vi "Format.vi"(6 "Statement":T1={"timestamp"=timestamp(0 s since 1904-01-01), "level"=enum."INFO", "sourceTag"="", "originVI"="", "message"=""}, 8 "error in (no error)":errorcluster, 11 "CSVLayout in":refnum<class "CSVLayout.lvclass">) -> (0 "error out":errorcluster, 3 "CSVLayout out":refnum<class "CSVLayout.lvclass">, 4 "FormattedLine":string)   [LabVIEW 2026, in "Lumberjack.lvlib" / "CSVLayout.lvclass"]
doc: "Override of Layout:Format. Emit the five Statement fields in column order, delimiter-joined, RFC 4180 quoted against the configured delimiter; timestamp as ISO 8601, level as its name (SRS-LMBR-012, SDD 5.4).\n\nTip: Emit one RFC 4180 delimited line (CSV/TSV) from a Statement."
uses:
  CSVLayout.lvclass
  TypeDefs/Statement.ctl
  TypeDefs/Severity.ctl
  CSVLayout.lvclass/CSVLayout.ctl
  Layout.lvclass/Layout.lvclass
  Lumberjack.lvlib
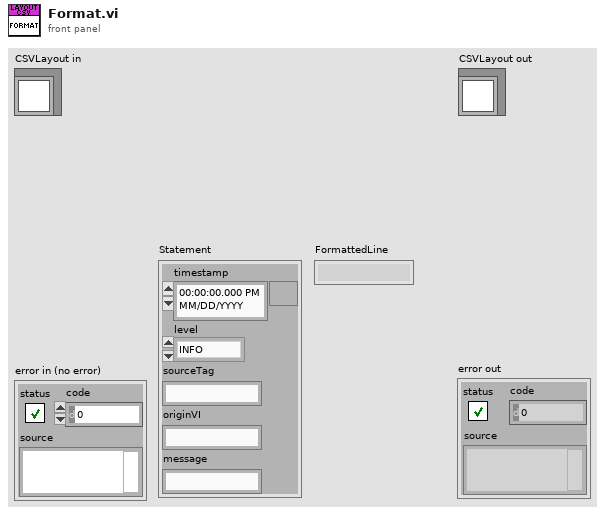
[diagram p1: front panel]
types:
  T1 = typedef "Lumberjack.lvlib/Statement.ctl" = cluster{"timestamp":timestamp, "level":T2, "sourceTag":string, "originVI":string, "message":string}
  T2 = typedef "Lumberjack.lvlib/Severity.ctl" = enum16{"OFF", "FATAL", "ERROR", "WARN", "INFO", "DEBUG", "TRACE", "ALL"}
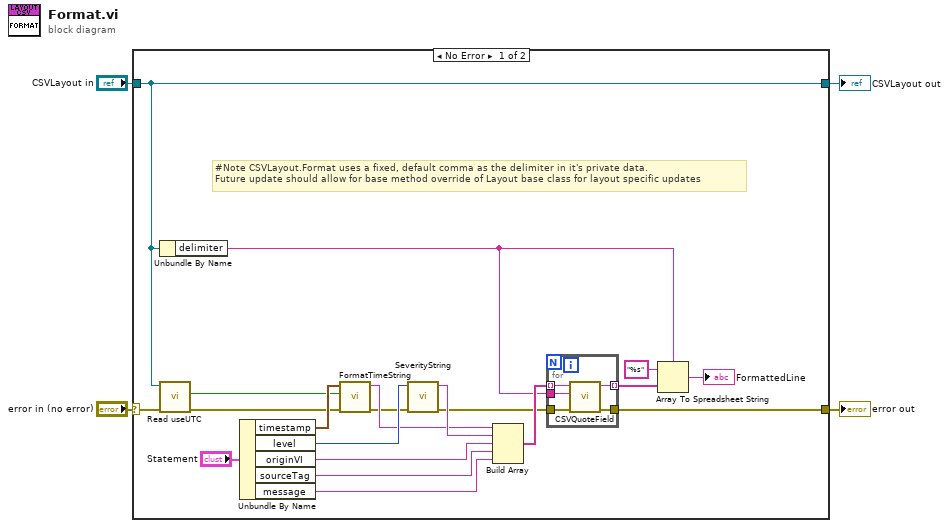
[diagram p0: block diagram]
diagram:
  n1 = case shown="No Error" "error in (no error)" {
    selector: "error in (no error)" -> [w24 w31]
    tunnel: [w16 w31] -> w4
    tunnel: [w11 w30] -> w3
    tunnel: "CSVLayout in" -> [w11 w30]
    frame No Error {
      # "#Note CSVLayout.Format uses a fixed, default comma as the delimiter in it's private data.\nFuture update should allow for base method override of Layout base class for layout specific updates"
      n2 = Unbundle By Name(w11) -> ("delimiter"=w15:string)
      n3 = call "Read useUTC.vi"("error in (no error)"=w24, "Layout in"=w11) -> ("error out"=w7:errorcluster, "useUTC"=w9:bool)  [unwired: 7 in, 1 out]
      n4 = Unbundle By Name("Statement") -> ("timestamp"=w10:timestamp, "level"=w22:T2, "originVI"=w20:string, "sourceTag"=w19:string, "message"=w18:string)
      n5 = call "FormatTimeString.vi"("error in (no error)"=w7, "useUTC"=w9, "timestamp"=w10) -> ("error out"=w6:errorcluster, "timeString"=w8:string)  [unwired: 7 in]
      n6 = call "SeverityString.vi"("error in (no error)"=w6, "Severity"=w22) -> ("error out"=w5:errorcluster, "SeverityString"=w21:string)  [unwired: 8 in]
      n7 = Build Array(w8, w21, w20, w19, w18) -> (w17:string[])
      n8 = for {
        tunnel: w17 -> [w29] mode=indexing
        tunnel: w15 -> [w28]
        tunnel: w5 -> [w27]
        tunnel: [w26] -> w16
        tunnel: [w25] -> w13 mode=indexing
        n9 = call "CSVQuoteField.vi"("error in (no error)"=w27, "delimiter"=w28, "field"=w29) -> ("error out"=w26:errorcluster, "quotedField"=w25:string)  [unwired: 7 in]
      }
      n10 = Array To Spreadsheet String(delimiter (Tab)=w15, array=w13, 3:"%s" ("format string")) -> (spreadsheet string=→"FormattedLine":string)
    }
    frame Error {
    }
  }
  "error out" <- w4
  "CSVLayout out" <- w3
